vi "Read Message Type.lvclass.vi"(8 "error in (no error)":errorcluster, 11 "User Receiver in":refnum<class "User Receiver.lvclass">) -> (0 "error out":errorcluster, 2 "Message Type.lvclass":refnum<class "Message Type.lvclass">, 3 "User Receiver out":refnum<class "User Receiver.lvclass">)   [LabVIEW 2023, in "User Receiver.lvclass"]
uses:
  User Receiver.lvclass
  User Receiver.lvclass/User Receiver.ctl
  Message Type/Message Type.lvclass
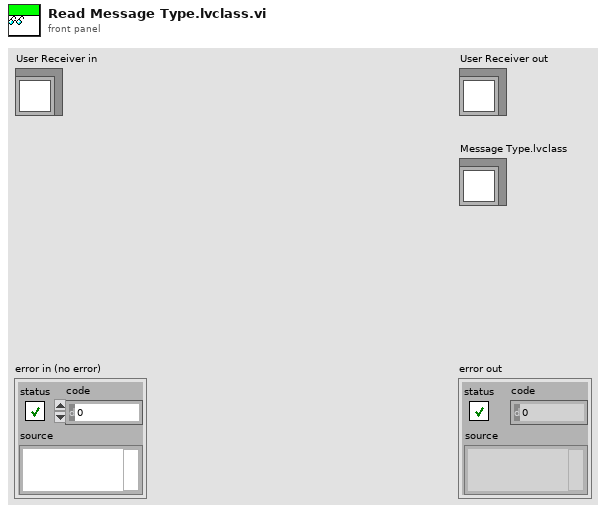
[diagram p1: front panel]
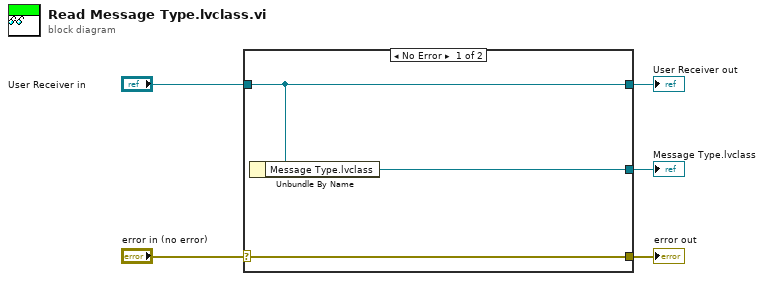
[diagram p0: block diagram]
diagram:
  n1 = case shown="No Error" "error in (no error)" {
    selector: "error in (no error)" -> [w8 w9]
    tunnel: [w8 w9] -> w4
    tunnel: [w7 w10] -> w2
    tunnel: "User Receiver in" -> [w7 w10]
    tunnel: [w6 _] -> w1
    frame No Error {
      n2 = Unbundle By Name(w7) -> ("Message Type.lvclass"=w6:refnum<class "Message Type.lvclass">)
    }
    frame Error {
    }
  }
  "error out" <- w4
  "User Receiver out" <- w2
  "Message Type.lvclass" <- w1
